vi "Abort Session.vi"(0 "session in":refnum<k21>, 11 "error in (no error)":errorcluster) -> (4 "session out":refnum<k21>, 15 "error out":errorcluster)   [LabVIEW 2020, in "SLSC.lvlib"]
doc: "Attempts to cancel a VI that blocks on network communications such as Connect to Devices or Add Network Chassis, making it wake up and return an error. After aborting the session, the session reference remains valid, but VIs that access network connections will return errors. To recover from an aborted session, close it and initialize a new one. Some operations, such as DNS lookups, cannot be aborted."
uses:
  <vilib>/SLSC/SLSC.lvlib
  nislsclvapi.dll
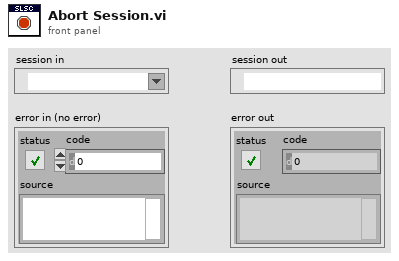
[diagram p1: front panel]
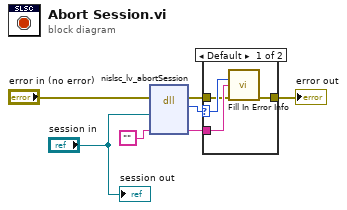
[diagram p0: block diagram]
diagram:
  n1 = dll-call lib="nislsclvapi.*" fn="nislsc_lv_abortSession"(error in="error in (no error)", "session"="session in", "extendedErrorInfo"="") -> (error out=w3:errorcluster, "return type"=w2:i32, "extendedErrorInfo"=w4:string)  [unwired: 5 in, 1 out]
  n2 = case shown="Default" w2 {
    selector: w2 -> [w11 _]
    tunnel: w4 -> [w10 _]
    tunnel: w3 -> [w9 w12]
    tunnel: [w8 w12] -> w1
    frame Default {
      n3 = call <vilib>:"Fill In Error Info.vi"("status code"=w11, "extended error info"=w10, "error in"=w9) -> ("error out"=w8:errorcluster)  [unwired: 12 in]
    }
    frame 0 {
    }
  }
  "error out" <- w1
  "session out" <- "session in"
